vi "Run Toolkit Integration Tests.vi"(8 "Error In":errorcluster) -> (0 "Error Out":errorcluster)   [LabVIEW 2018, in "Scripts.lvlib"]
uses:
  Scripts.lvlib
  tests/Toolkit/Integration/Integration.lvlib
  <vilib>/addons/_JKI Toolkits/Caraya/classes/Test/Test.lvclass
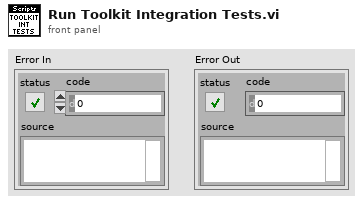
[diagram p1: front panel]
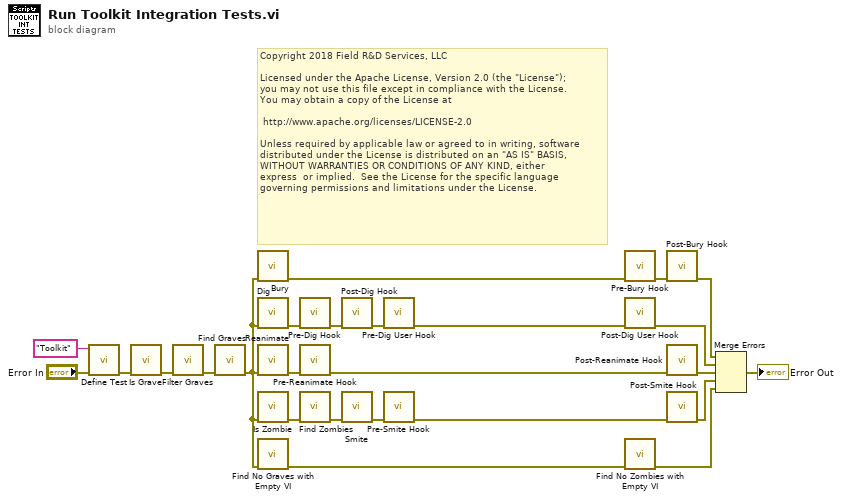
[diagram p0: block diagram]
diagram:
  # "Copyright 2018 Field R&D Services, LLC\n\nLicensed under the Apache License, Version 2.0 (the \"License\");\nyou may not use this file except in compliance with the License.\nYou may obtain a copy of the License at\n\n\thttp://www.apache.org/licenses/LICENSE-2.0\n\nUnless required by applicable law or agreed to in writing, software\ndistributed under the License is distributed on an \"AS IS\" BASIS,\nWITHOUT WARRANTIES OR CONDITIONS OF ANY KIND, either \nexpress  or implied.  See the License for the specific language \ngoverning permissions and limitations under the License."
  n1 = call <vilib>:"Define Test.vi"("error in (no error)"="Error In", "Label (VI Title)"="Toolkit") -> ("error out"=w22:errorcluster)  [unwired: 9 in]
  n2 = call "Is Grave.vi"("Error In"=w22) -> ("Error Out"=w24:errorcluster)  [unwired: 10 in]
  n3 = call "Filter Graves.vi"("Error In"=w24) -> ("Error Out"=w23:errorcluster)  [unwired: 10 in]
  n4 = call "Find Graves.vi"("Error In"=w23) -> ("Error Out"=w16:errorcluster)  [unwired: 10 in]
  n5 = call "Bury.vi"("Error In"=w16) -> ("Error Out"=w12:errorcluster)  [unwired: 10 in]
  n6 = call "Dig.vi"("Error In"=w16) -> ("Error Out"=w18:errorcluster)  [unwired: 10 in]
  n7 = call "Reanimate.vi"("Error In"=w16) -> ("Error Out"=w9:errorcluster)  [unwired: 10 in]
  n8 = call "Is Zombie.vi"("Error In"=w16) -> ("Error Out"=w25:errorcluster)  [unwired: 10 in]
  n9 = call "Find No Graves with Empty VI.vi"("Error In"=w16) -> ("Error Out"=w14:errorcluster)  [unwired: 10 in]
  n10 = call "Pre-Dig Hook.vi"("Error In"=w18) -> ("Error Out"=w17:errorcluster)  [unwired: 10 in]
  n11 = call "Pre-Reanimate Hook.vi"("Error In"=w9) -> ("Error Out"=w8:errorcluster)  [unwired: 10 in]
  n12 = call "Find Zombies.vi"("Error In"=w25) -> ("Error Out"=w15:errorcluster)  [unwired: 10 in]
  n13 = call "Post-Dig Hook.vi"("Error In"=w17) -> ("Error Out"=w3:errorcluster)  [unwired: 10 in]
  n14 = call "Smite.vi"("Error In"=w15) -> ("Error Out"=w6:errorcluster)  [unwired: 10 in]
  n15 = call "Pre-Dig User Hook.vi"("Error In"=w3) -> ("Error Out"=w2:errorcluster)  [unwired: 10 in]
  n16 = call "Pre-Smite Hook.vi"("Error In"=w6) -> ("Error Out"=w5:errorcluster)  [unwired: 10 in]
  n17 = call "Pre-Bury Hook.vi"("Error In"=w12) -> ("Error Out"=w11:errorcluster)  [unwired: 10 in]
  n18 = call "Post-Dig User Hook.vi"("Error In"=w2) -> ("Error Out"=w1:errorcluster)  [unwired: 10 in]
  n19 = call "Find No Zombies with Empty VI.vi"("Error In"=w14) -> ("Error Out"=w13:errorcluster)  [unwired: 10 in]
  n20 = call "Post-Bury Hook.vi"("Error In"=w11) -> ("Error Out"=w10:errorcluster)  [unwired: 10 in]
  n21 = call "Post-Reanimate Hook.vi"("Error In"=w8) -> ("Error Out"=w7:errorcluster)  [unwired: 10 in]
  n22 = call "Post-Smite Hook.vi"("Error In"=w5) -> ("Error Out"=w4:errorcluster)  [unwired: 10 in]
  n23 = Merge Errors(w10, w1, w7, w4, w13) -> (→"Error Out":errorcluster)
